vi "RTS Door Ops Timer.vi"(8 "Error In":errorcluster, 10 "Door Open Delay(sec)":dbl, 11 "Routine Complete":bool) -> (0 "Error Out":errorcluster, 1 "Elapsed Time (sec)":dbl, 3 "Time has Elapsed":bool)   [LabVIEW 2016]
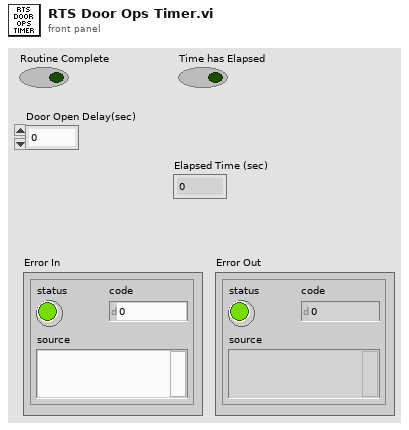
[diagram p1: front panel]
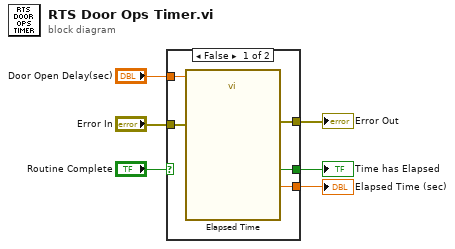
[diagram p0: block diagram]
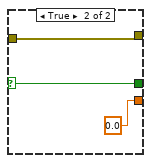
[diagram p2: hidden frame]
diagram:
  n1 = case shown="False" "Routine Complete" {
    selector: "Routine Complete" -> [_ w14]
    tunnel: [w11 w14] -> w6
    tunnel: "Door Open Delay(sec)" -> [w10 _]
    tunnel: [w9 0.0 ("Elapsed Time (s)")] -> w5
    tunnel: "Error In" -> [w8 w12]
    tunnel: [w7 w12] -> w1
    frame False {
      n2 = call "Elapsed Time"("Time Target (s)"=w10, "error in (no error)"=w8) -> ("Elapsed Time (s)"=w9:dbl, "Time has Elapsed"=w11:bool, "error out"=w7:errorcluster)  [unwired: 10 in, 5 out]
    }
    frame True {
    }
  }
  "Elapsed Time (sec)" <- w5
  "Time has Elapsed" <- w6
  "Error Out" <- w1
